vi "MeasAction.vi"(8 "error in (no error)":errorcluster caption="entrée d'erreur (pas d'erreur)", 9 "CurvePointIndex":i32, 10 "AllPointIndex":i32, 11 "GenData In":refnum<class "Tools.lvclass"> caption="DNL_LabVIEW Object in") -> (0 "error out":errorcluster caption="sortie d'erreur", 2 "MeasDatOut":dbl[](array[numeric]), 3 "GenData Out":refnum<class "Tools.lvclass"> caption="DNL_LabVIEW Object out")   [LabVIEW 2019, in "Tools.lvclass"]
uses:
  Tools.lvclass
  C:/Programmes Labview/LabScanV1A/DevicesClass/BaseDevice/BaseDevice.lvclass
  Tools.lvclass/Tools.ctl
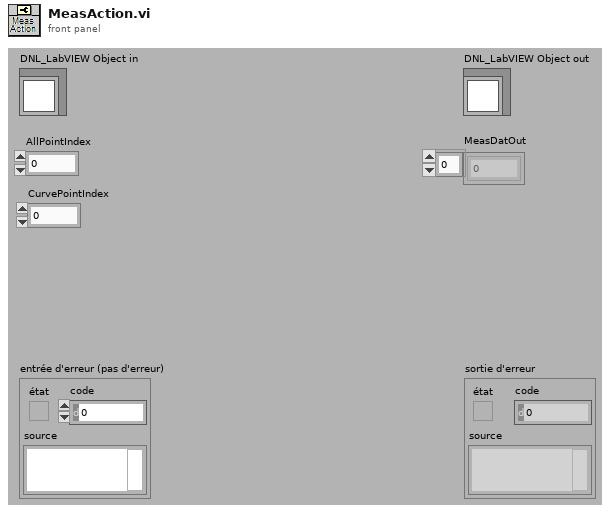
[diagram p1: front panel]
types:
  T1 = typedef "Tools.lvclass/Tools_Func.ctl" = enum16{"Courbe 1 (Arb)", "Courbe 2 (Arb)", "Courbe 3 (Arb)", "Courbe 123 (Arb,Arb,Arb)", "Scan Pos (Arb)", "Indice de Point (Points)", "AbsTime (ms)", "Minuteur (s)", "Panneaux Infos (Na)", "Délais (ms)", "RandwithDbind(Arb)", "RandomNum (Arb)", "Multisweep (Sw)", "ScanTime (s)"}
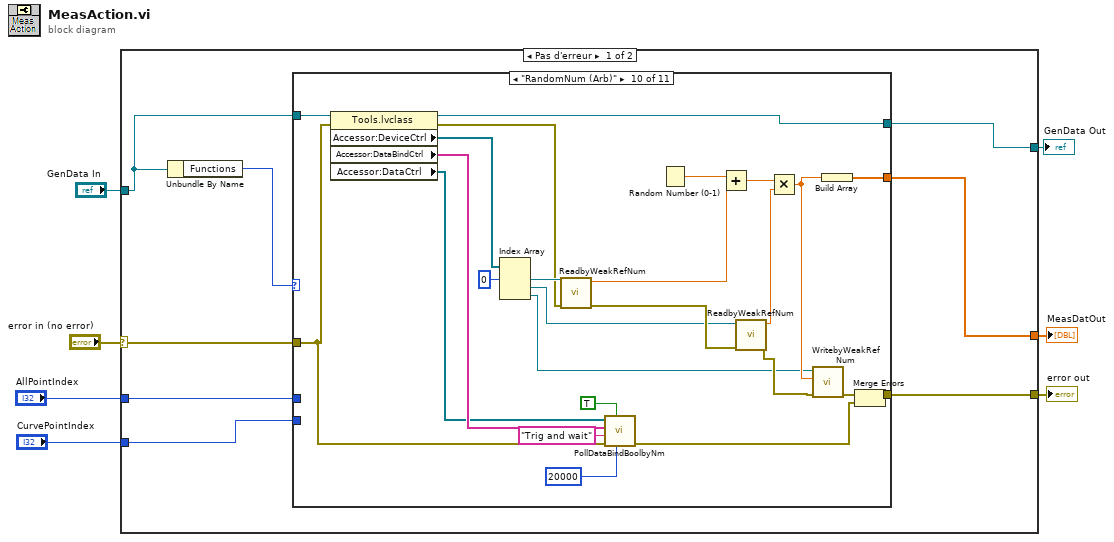
[diagram p0: block diagram]
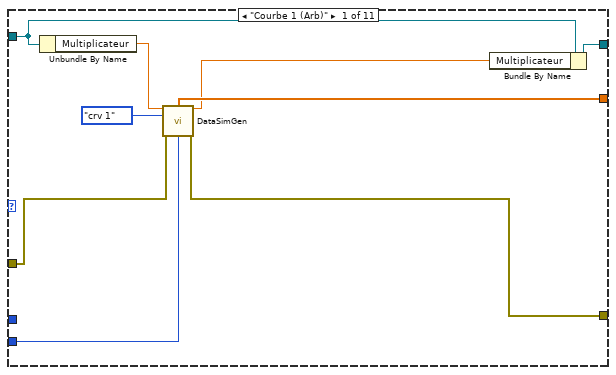
[diagram p2: hidden frame]
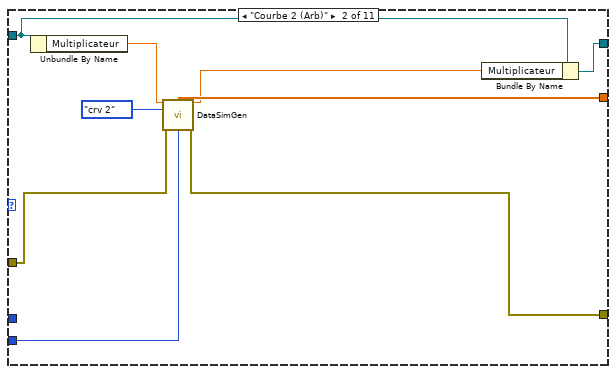
[diagram p3: hidden frame]
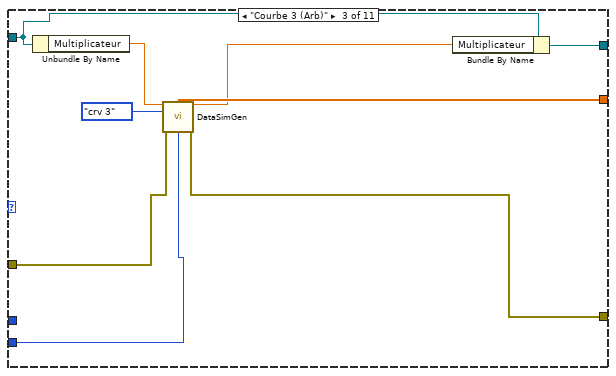
[diagram p4: hidden frame]
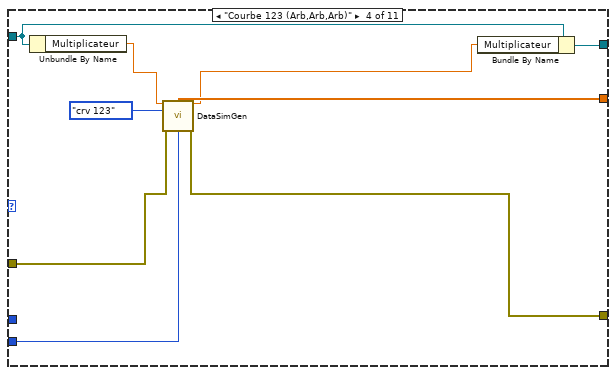
[diagram p5: hidden frame]
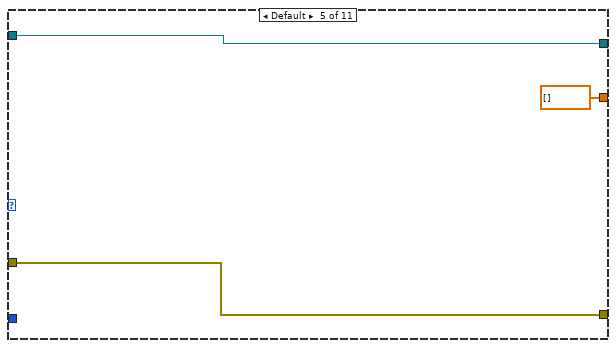
[diagram p6: hidden frame]
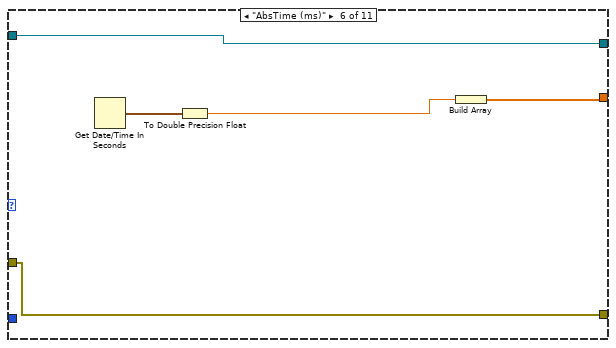
[diagram p7: hidden frame]
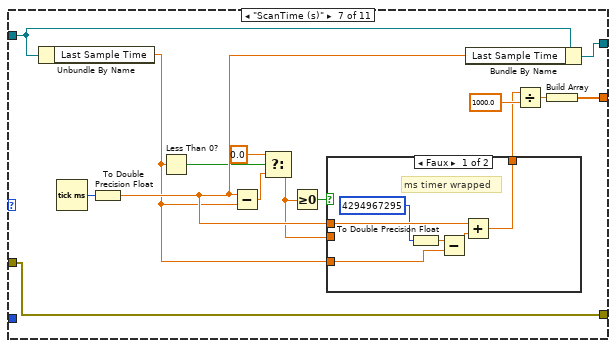
[diagram p8: hidden frame]
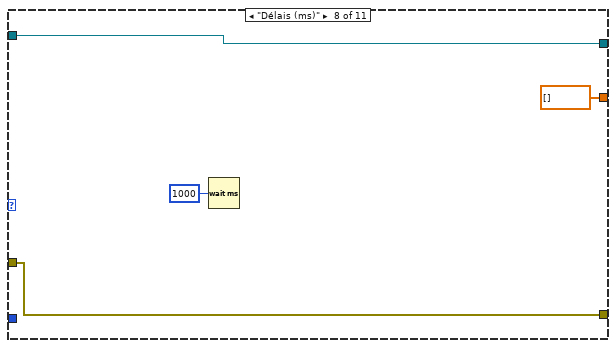
[diagram p10: hidden frame]
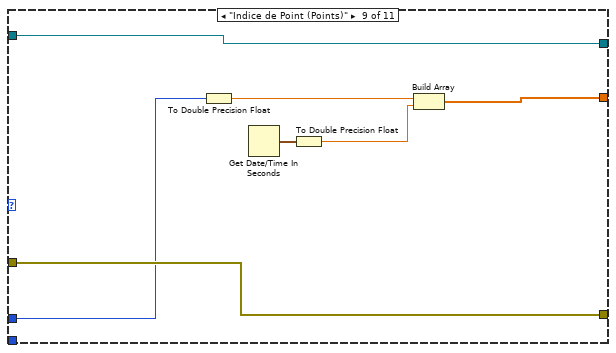
[diagram p11: hidden frame]
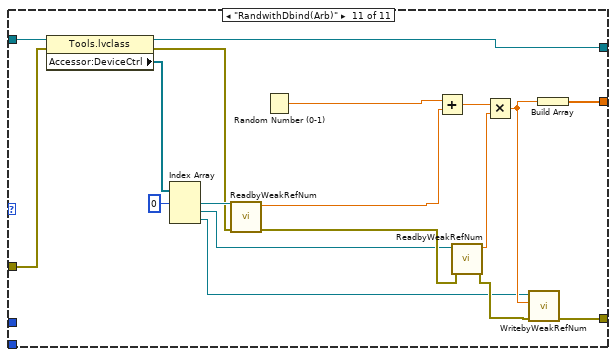
[diagram p12: hidden frame]
diagram:
  n1 = case shown="Pas d'erreur" "error in (no error)" {
    selector: "error in (no error)" -> [w11 w136]
    tunnel: "GenData In" -> [w9 w137]
    tunnel: [w8 w137] -> w5
    tunnel: "AllPointIndex" -> [w15 _]
    tunnel: [w14 w136] -> w3
    tunnel: [w13 _] -> w2
    tunnel: "CurvePointIndex" -> [w10 _]
    frame No Error {
      n2 = Unbundle By Name(w9) -> ("Functions"=w12:T1)
      n3 = case shown="\"RandomNum (Arb)\"" w12 {
        tunnel: w15 -> [_ _ _ _ _ _ _ _ w89 _ _]
        tunnel: [w24 w33 w42 w51 w53 w56 w73 w84 w92 w94 w122] -> w14
        tunnel: [w22 w31 w40 w49 dbl[] [] ("Outputs") w57 w74 dbl[] [] ("Outputs") w90 w117 w135] -> w13
        tunnel: w11 -> [w21 w30 w39 w48 w53 w56 w73 w84 w92 w97 w133]
        tunnel: w10 -> [w20 w29 w38 w47 _ _ _ _ _ _ _]
        tunnel: w9 -> [w18 w25 w37 w43 w52 w55 w71 w82 w88 w102 w119]
        tunnel: [w19 w27 w36 w44 w52 w55 w72 w82 w88 w101 w118] -> w8
        frame "Courbe 1 (Arb)" {
          n4 = Unbundle By Name(w18) -> ("Multiplicateur"=w17:dbl)
          n5 = call <userlib>:"DataSimGen.vi"("multiplicateur"=w17, "Données"=enum16{"crv 1", "crv 2", "crv 3", "crv 123"}."crv 1", "error in (no error)"=w21, "IndicePoint"=w20) -> ("Outputs"=w22:dbl[], "multiplicateur out"=w16:dbl, "error out"=w24:errorcluster)  [unwired: 8 in, 1 out]
          n6 = Bundle By Name(cluster=w18, "Multiplicateur"=w16) -> (w19:refnum<class "Tools.lvclass">)
        }
        frame "Courbe 2 (Arb)" {
          n7 = Unbundle By Name(w25) -> ("Multiplicateur"=w26:dbl)
          n8 = call <userlib>:"DataSimGen.vi"("multiplicateur"=w26, "Données"=enum16{"crv 1", "crv 2", "crv 3", "crv 123"}."crv 2", "error in (no error)"=w30, "IndicePoint"=w29) -> ("Outputs"=w31:dbl[], "multiplicateur out"=w28:dbl, "error out"=w33:errorcluster)  [unwired: 8 in, 1 out]
          n9 = Bundle By Name(cluster=w25, "Multiplicateur"=w28) -> (w27:refnum<class "Tools.lvclass">)
        }
        frame "Courbe 3 (Arb)" {
          n10 = Unbundle By Name(w37) -> ("Multiplicateur"=w34:dbl)
          n11 = call <userlib>:"DataSimGen.vi"("multiplicateur"=w34, "Données"=enum16{"crv 1", "crv 2", "crv 3", "crv 123"}."crv 3", "error in (no error)"=w39, "IndicePoint"=w38) -> ("Outputs"=w40:dbl[], "multiplicateur out"=w35:dbl, "error out"=w42:errorcluster)  [unwired: 8 in, 1 out]
          n12 = Bundle By Name(cluster=w37, "Multiplicateur"=w35) -> (w36:refnum<class "Tools.lvclass">)
        }
        frame "Courbe 123 (Arb,Arb,Arb)" {
          n13 = Unbundle By Name(w43) -> ("Multiplicateur"=w46:dbl)
          n14 = call <userlib>:"DataSimGen.vi"("multiplicateur"=w46, "Données"=enum16{"crv 1", "crv 2", "crv 3", "crv 123"}."crv 123", "error in (no error)"=w48, "IndicePoint"=w47) -> ("Outputs"=w49:dbl[], "multiplicateur out"=w45:dbl, "error out"=w51:errorcluster)  [unwired: 8 in, 1 out]
          n15 = Bundle By Name(cluster=w43, "Multiplicateur"=w45) -> (w44:refnum<class "Tools.lvclass">)
        }
        frame Default {
        }
        frame "AbsTime (ms)" {
          n16 = Get Date/Time In Seconds() -> (seconds since 1Jan1904=w59:timestamp)
          n17 = To Double Precision Float(number=w59) -> (double precision float=w58:dbl)
          n18 = Build Array(w58) -> (w57:dbl[])
        }
        frame "ScanTime (s)" {
          n19 = Unbundle By Name(w71) -> ("Last Sample Time"=w64:dbl)
          n20 = Tick Count (ms)() -> (millisecond timer value=w70:u32)
          n21 = To Double Precision Float(number=w70) -> (double precision float=w65:dbl)
          n22 = Less Than 0?(x=w64) -> (x < 0?=w63:bool)
          n23 = Subtract(x=w65, y=w64) -> (x-y=w61:dbl)
          n24 = Select(t=0.0, s=w63, f=w61) -> (s? t:f=w60:dbl)
          n25 = Greater Or Equal To 0?(x=w60) -> (x >= 0?=w67:bool)
          n26 = case shown="Faux" w67 {
            tunnel: w60 -> [_ w81]
            tunnel: [w77 w81] -> w66
            tunnel: w64 -> [w80 _]
            tunnel: w65 -> [w78 _]
            frame False {
              # "ms timer wrapped"
              n27 = To Double Precision Float(number=u32 4294967295 ("x")) -> (double precision float=w75:dbl)
              n28 = Subtract(x=w75, y=w80) -> (x-y=w79:dbl)
              n29 = Add(x=w78, y=w79) -> (x+y=w77:dbl)
            }
            frame True {
            }
          }
          n30 = Bundle By Name(cluster=w71, "Last Sample Time"=w65) -> (w72:refnum<class "Tools.lvclass">)
          n31 = Divide(x=w66, y=1000.0) -> (x/y=w69:dbl)
          n32 = Build Array(w69) -> (w74:dbl[])
        }
        frame "Délais (ms)" {
          n33 = Wait (ms)(milliseconds to wait=u32 1000 ("attente (ms)")) -> ()  [unwired: 1 out]
        }
        frame "Indice de Point (Points)" {
          n34 = To Double Precision Float(number=w89) -> (double precision float=w91:dbl)
          n35 = Get Date/Time In Seconds() -> (seconds since 1Jan1904=w87:timestamp)
          n36 = To Double Precision Float(number=w87) -> (double precision float=w86:dbl)
          n37 = Build Array(w91, w86) -> (w90:dbl[])
        }
        frame "RandomNum (Arb)" {
          n38 = property class="Tools.lvclass"(reference=w102, error in=w97) -> (reference out=w101:refnum<class "Tools.lvclass">, error out=w112:errorcluster, "Accessor:DeviceCtrl"=w116:refnum<vi>[], "Accessor:DataBindCtrl"=w100:string[], "Accessor:DataCtrl"=w99:refnum<vi>[])
          n39 = Index Array(array=w116, index #1=0 ("indice")) -> (element #1=w113:refnum<vi>, element #2=w109:refnum<vi>, element #3=w103:refnum<vi>)  [unwired: 2 in]
          n40 = call <userlib>:"ReadbyWeakRefNum.vi"("error in"=w112, "Control Ref"=w113) -> ("error out"=w110:errorcluster, "Valeur"=w111:dbl)  [unwired: 8 in]
          n41 = call <userlib>:"PollDataBindBoolbyNm.vi"("Timeout(ms)"=20000, "Valeur"=TRUE, "error in"=w97, "TargetName"="Trig and wait", "DataBindCtrlNm"=w100, "Control Ref"=w99) -> ("error out"=w93:errorcluster)  [unwired: 4 in, 1 out]
          n42 = Random Number (0-1)() -> (number: 0 to 1=w114:dbl)
          n43 = Add(x=w114, y=w111) -> (x+y=w108:dbl)
          n44 = call <userlib>:"ReadbyWeakRefNum.vi"("error in"=w110, "Control Ref"=w109) -> ("error out"=w106:errorcluster, "Valeur"=w107:dbl)  [unwired: 8 in]
          n45 = Multiply(x=w108, y=w107) -> (x*y=w104:dbl)
          n46 = call <userlib>:"WritebyWeakRefNum.vi"("error in"=w106, "Valeur"=w104, "Control Ref"=w103) -> ("error out"=w105:errorcluster)  [unwired: 8 in]
          n47 = Build Array(w104) -> (w117:dbl[])
          n48 = Merge Errors(w105, w93) -> (w94:errorcluster)
        }
        frame "RandwithDbind(Arb)" {
          n49 = property class="Tools.lvclass"(reference=w119, error in=w133) -> (reference out=w118:refnum<class "Tools.lvclass">, error out=w129:errorcluster, "Accessor:DeviceCtrl"=w134:refnum<vi>[])
          n50 = Index Array(array=w134, index #1=0 ("indice")) -> (element #1=w130:refnum<vi>, element #2=w126:refnum<vi>, element #3=w120:refnum<vi>)  [unwired: 2 in]
          n51 = call <userlib>:"ReadbyWeakRefNum.vi"("error in"=w129, "Control Ref"=w130) -> ("error out"=w127:errorcluster, "Valeur"=w128:dbl)  [unwired: 8 in]
          n52 = Random Number (0-1)() -> (number: 0 to 1=w131:dbl)
          n53 = Add(x=w131, y=w128) -> (x+y=w125:dbl)
          n54 = call <userlib>:"ReadbyWeakRefNum.vi"("error in"=w127, "Control Ref"=w126) -> ("error out"=w123:errorcluster, "Valeur"=w124:dbl)  [unwired: 8 in]
          n55 = Multiply(x=w125, y=w124) -> (x*y=w121:dbl)
          n56 = call <userlib>:"WritebyWeakRefNum.vi"("error in"=w123, "Valeur"=w121, "Control Ref"=w120) -> ("error out"=w122:errorcluster)  [unwired: 8 in]
          n57 = Build Array(w121) -> (w135:dbl[])
        }
      }
    }
    frame Error {
    }
  }
  "error out" <- w3
  "GenData Out" <- w5
  "MeasDatOut" <- w2
